vi "FPGAmain_5782_IQ_PID_2.vi"() -> ()   [LabVIEW 2018]
uses:
  FPGA/DataMode.ctl
  FPGA/Input_5782/5782_Fast_PID_states.ctl
  FPGA/Feed forward/FeedForwardState.ctl
  <vilib>/Platform/TimedLoop/XDataNode/timing_clust.ctl
  <vilib>/Platform/TimedLoop/XDataNode/nitl_modes.ctl
  <vilib>/Platform/TimedLoop/XDataNode/wakeup.ctl
  <vilib>/rvi/Emulation/niFpgaSctlEmulationGetInTimedLoop.vi
  <vilib>/rvi/Emulation/niFpgaEmulationReportErrorSimple.vi
  <vilib>/rvi/Emulation/niFpgaGetClockAttributes.vi
  <vilib>/rvi/Emulation/niFpgaCriticalErrorInLSC.vi
  <vilib>/rvi/Emulation/niFpgaProcessEmulError.vi
  <vilib>/rvi/Emulation/niFpgaEmulationIsFPGAContextNoSignature.vi
  <vilib>/rvi/errors/niFpgaSetErrorForExecOnDevCompSimple.vi
  <vilib>/rvi/eio/common/nirviEmuReportErrorAndStop.vi
  <vilib>/rvi/DataTransferAndStorage/Container/Common/niFpgaContainerGetUniqueNameForEmu.vi
  <vilib>/rvi/FIFO/Fifo_Resource/nirvififoEmulationSetSize.vi
  <vilib>/rvi/FIFO/Fifo_Resource/nirviFifoEmulationQueueMgr.vi
  <instcachedir>/0/nirviFifoEmulationQueueMgr_E5CAEC123FF24DC58D834DCA3CDAA9B5.lvgen/nirviFifoEmulationQueueMgr_E5CAEC123FF24DC58D834DCA3CDAA9B5_015.vi
  <vilib>/rvi/FIFO/Fifo_Resource/nirvififoEmulationDetermineInputValidOut.vi
  <vilib>/rvi/FIFO/Fifo_Resource/nirvififoEmulationCreateLock.vi
  <vilib>/rvi/FIFO/Fifo_Resource/nirvififoEmulationObtainLock.vi
  <vilib>/rvi/FIFO/Fifo_Resource/nirvififoEmulationReleaseLock.vi
  <vilib>/rvi/occurrence/nirviWaitOnOccurrenceBase.vi
  <vilib>/rvi/errors/nirviReportUnexpectedCaseInternalError.vi
  <vilib>/rvi/errors/nirviReportUnexpectedCaseInternalError (U32).vi
  <vilib>/rvi/Memory/Memory_Emulation/niFpgaMemoryEmulationCacheClearOnFirstRun.vi
  <vilib>/rvi/Memory/Memory_Emulation/nirvimemoryEmulationManagerCache_MakeExclusive.vi
  <vilib>/rvi/Memory/Memory_Emulation/niFpgaMemoryEmulationValidateCache.vi
  <vilib>/rvi/Memory/Memory_Emulation/nirvimemoryEmulationManagerCache_InsertValue.vi
  <vilib>/Utility/error.llb/Clear Errors.vi
  <vilib>/rvi/Memory/Memory_Emulation/nirvimemoryEmulationManagerCache_ReleaseExclusive.vi
  <vilib>/rvi/Memory/Memory_Emulation/nirvimemoryEmulationManagerCache_GetValue.vi
  <vilib>/rvi/Memory/Memory_Emulation/nirvimemoryEmulationManagerCache_SetValue.vi
  <vilib>/rvi/eio/common/nirviEmuTemplateMethod_errors.vi
  <instcachedir>/0/nirviFifoEmulationQueueMgr_E5CAEC123FF24DC58D834DCA3CDAA9B5.lvgen/nirviFifoEmulationQueueMgr_E5CAEC123FF24DC58D834DCA3CDAA9B5_018.vi
  <vilib>/rvi/interface/RandomDataEmulation/niFpgaRandomDataHandleErrors.vi
  <instcachedir>/0/nirviFifoEmulationQueueMgr_E5CAEC123FF24DC58D834DCA3CDAA9B5.lvgen/nirviFifoEmulationQueueMgr_E5CAEC123FF24DC58D834DCA3CDAA9B5_003.vi
  <instcachedir>/0/nirviFifoEmulationQueueMgr_E5CAEC123FF24DC58D834DCA3CDAA9B5.lvgen/nirviFifoEmulationQueueMgr_E5CAEC123FF24DC58D834DCA3CDAA9B5_017.vi
  <vilib>/rvi/interface/RandomDataEmulation/nirviRandomDataMultiElementFPGAFIFO.vi
  <instcachedir>/0/nirviRandomDataMultiElementFPGAFIFO_6740B454F3C245F78F76ED91F73FD8DB.lvgen/nirviRandomDataMultiElementFPGAFIFO_6740B454F3C245F78F76ED91F73FD8DB_000.vi
  <instrlib>/_niInstr/Basic Elements/v1/FPGA/Private/Count Down U8.vi
  <vilib>/rvi/Memory/Memory_Emulation/nirvimemoryFastEmulation.vi
  <vilib>/rvi/Memory/Memory_Emulation/nirvimemoryEmulation.vi
  <vilib>/Platform/TimedLoop/XDataNode/XDataNode.xnode
  <vilib>/rvi/FXPMathLib/FxpInterpret/XNode/nifxpmath_Interpret.xnode
  <vilib>/rvi/DataTransferAndStorage/Container/XNode/niFpgaContainer.xnode
  <vilib>/rvi/FIFO/Fifo_Resource/nirvififoEmulationWrite.vi
  <vilib>/rvi/DataTransferAndStorage/Register/Emulation/niFpgaRegisterEmulation.vi
  <vilib>/eio/EIONode/EIONode.xnode
  <vilib>/rvi/FIFO/Fifo_Resource/nirvififoEmulationRead.vi
  <vilib>/rvi/interface/RandomDataEmulation/nirviRandomDataFpgaReadWriteTemplate.vi
  <vilib>/rvi/interface/RandomDataEmulation/nirviRandomDataFpgaMultiElementTemplate.vi
  <vilib>/Platform/TimedLoop/XDataNode/XDNodeRunTimeDep.lvlib
  <instrlib>/_niInstr/Basic Elements/v1/FPGA/niInstr Basic Elements v1 FPGA.lvlib
panel:
  in  "Load FF":bool
  in  "Clear feedback buffers":bool
  in  "FF buffers manual":bool
  in  "Full speed transfer":bool
  in  "IO Module\\AO Data Sync":bool=TRUE
  in  "IO Module\\SPI Write Data":u16
  out "IO Module\\SPI Read Data":u8
  in  "IO Module\\SPI Read":bool
  in  "IO Module\\SPI Write":bool
  in  "IO Module\\SPI Address":u16
  in  "IO Module\\SPI Device":u8
  out "IO Module\\SPI Idle":bool
  in  "AM phase":fxp<+,64,64>
  in  "User Command Commit":bool
  in  "User Command":u8
  out "User Command Idle":bool
  out "User Command Status":u8
  in  "User Data 0":u8
  in  "User Data 1":u8
  out "PLL Locked":bool
  out "User Error":bool
  out "Configured?":bool
  in  "Continuous":bool
  in  "Record length":u16=4000 caption="Samples Per Trigger" min=1 step=1
  in  "Trigger Acquisition":bool
  out "IO Module\\Trigger Input":bool
  in  "Acquisition running":bool
  in  "Phase output":fxp<+,64,64>[](array[numeric])=[0.0, 0.0, 0.0, 0.0]
  in  "Simulated phase":fxp<+,64,64>[](array[numeric])=[0.0, 0.0]
  in  "Mode":T1
  in  "Phase input":fxp<+,64,64>[](array[numeric])=[0.0, 0.0, 0.0, 0.0, 0.0, 0.0, 0.0, 0.0, 0.0, 0.0, 0.0, 0.0, 0.0, 0.0, 0.0, 0.0]
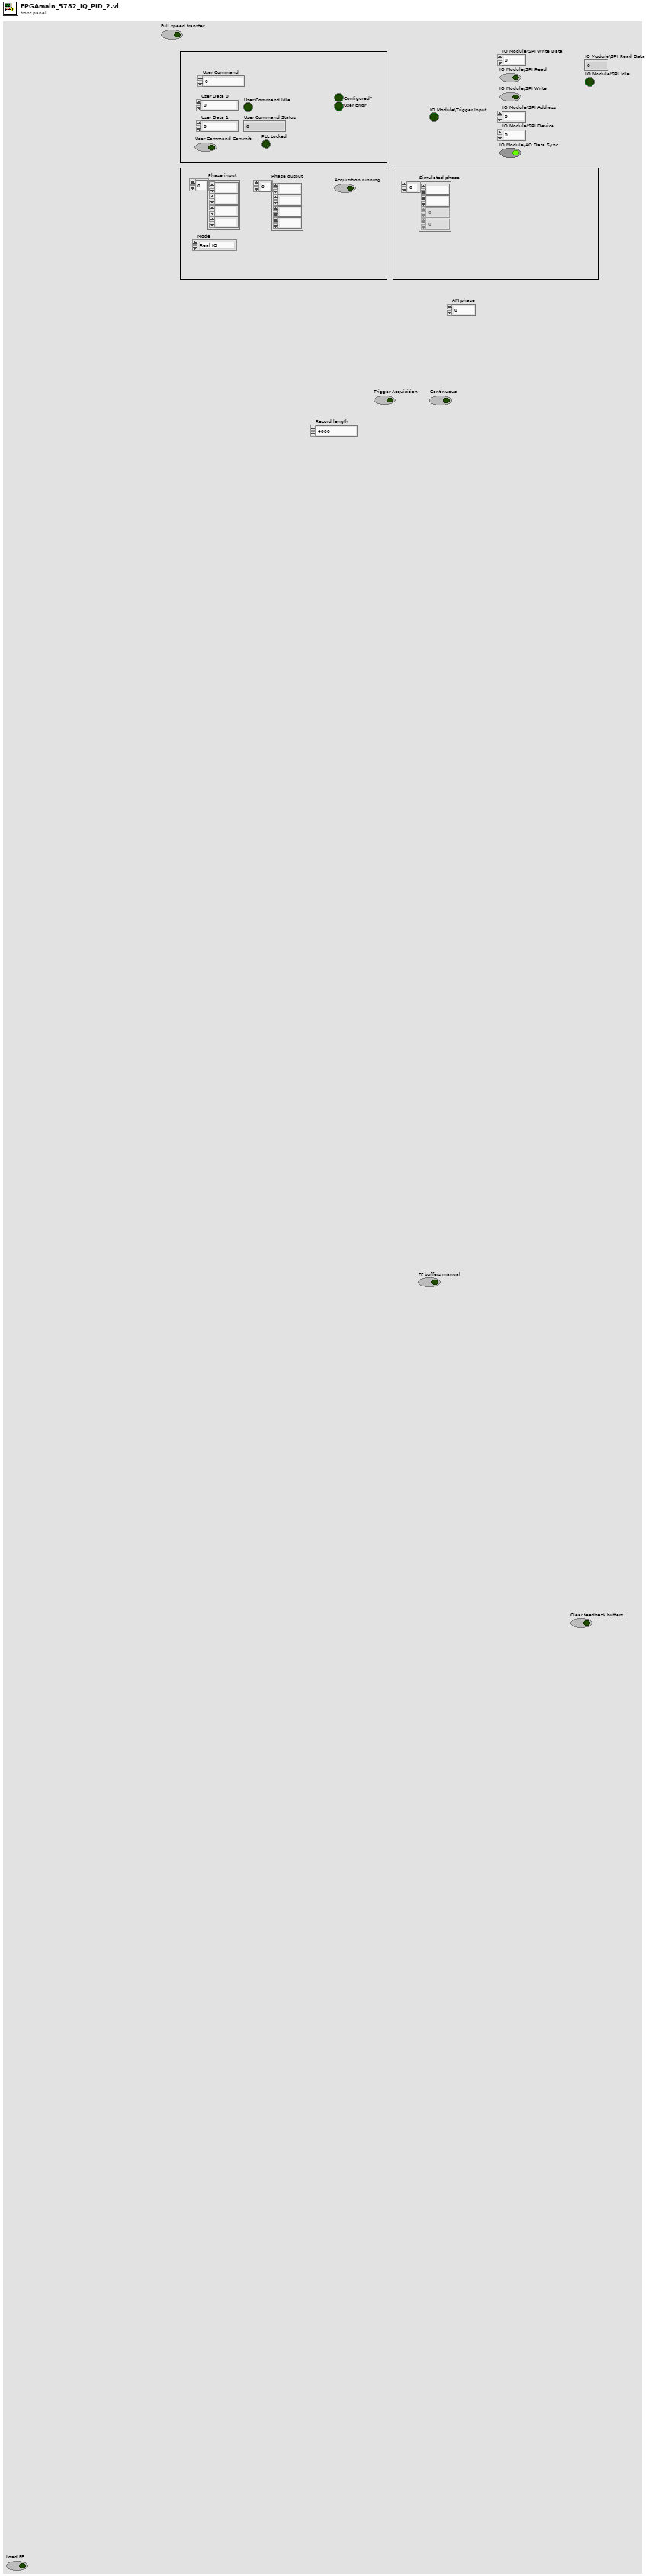
[diagram p1: front panel]
types:
  T1 = typedef "DataMode.ctl" = enum16{"Real IO", "Simulated"}
  T2 = typedef "FeedForwardState.ctl" = enum16{"Idle", "Wait for trigger", "Read FF", "Clear FF", "Wait for reset"}
  T3 = typedef "5782_Fast_PID_states.ctl" = enum8{"Wait for trigger", "Acquisition", "Send record length", "Wait for output", "Quiet period"}
  T4 = typedef "XDNodeRunTimeDep.lvlib/timing_clust.ctl" = cluster{"Expected End [f-1]":u64, "Actual End [f-1]":u64, "Finished Late? [f-1]":bool, "Expected End [i-1]":u64, "Actual End [i-1]":u64, "Finished Late? [i-1]":bool, "Expected Start [i]":u64, "Actual Start [i]":u64, "Expected Start [f]":u64, "Actual Start [f]":u64, "Source Name":string, "Structure Name":string, "Period":i64, "Deadline":i64, "Offset":i64, "Start":i64, "Priority":i32, "Timeout":i32, "Mode":T5, "Wakeup Reason":T6, "Error":errorcluster, "Source Type":string, "Secondary Source Type":string, "Global End Time":u64, "Global Start Time":u64, "Frame Duration":u64, "Iteration Duration":u64, "Assigned CPU":i32, "I/O Scan Engine Mode":u32}
  T5 = typedef "XDNodeRunTimeDep.lvlib/nitl_modes.ctl" = enum32{"No Change", "Process missed periods, maintain original phase", "Discard missed periods, maintain original phase", "Process missed periods, ignore original phase", "Discard missed periods, ignore original phase"}
  T6 = typedef "XDNodeRunTimeDep.lvlib/wakeup.ctl" = enum32{"Normal", "Aborted", "Asynchronous wakeup", "Timing source error", "Timed loop error", "Timeout"}
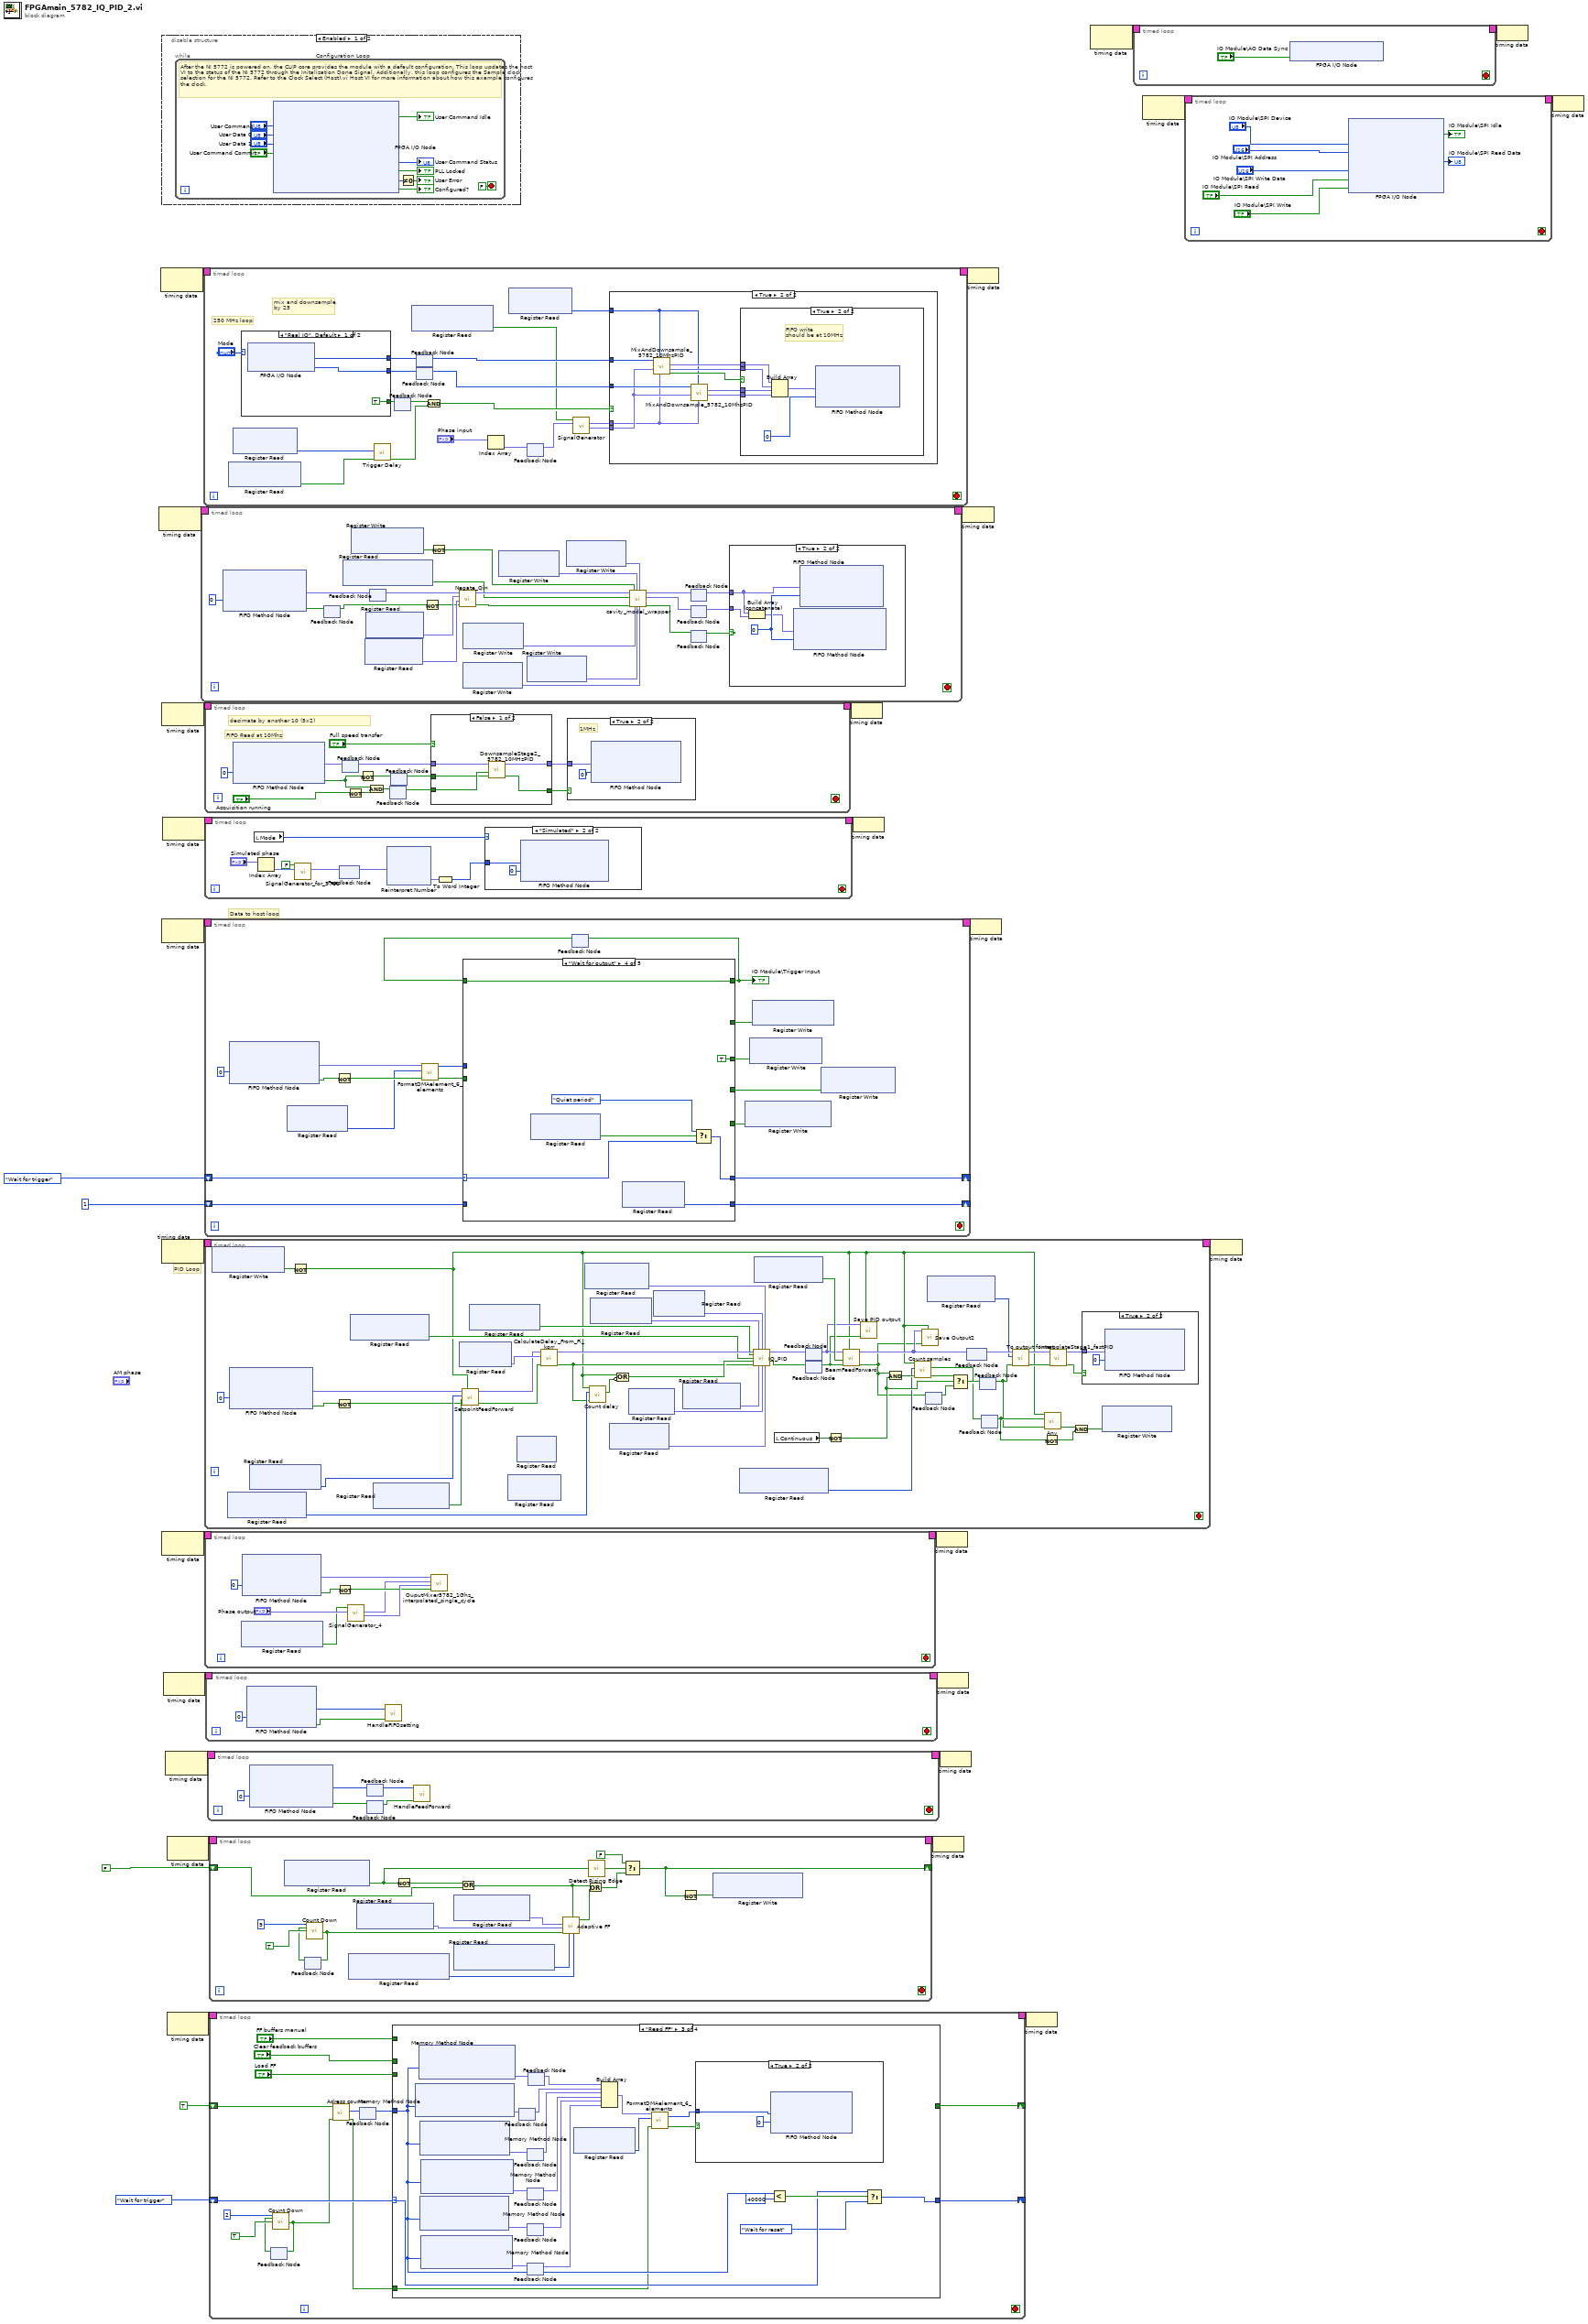
[diagram p0: block diagram]
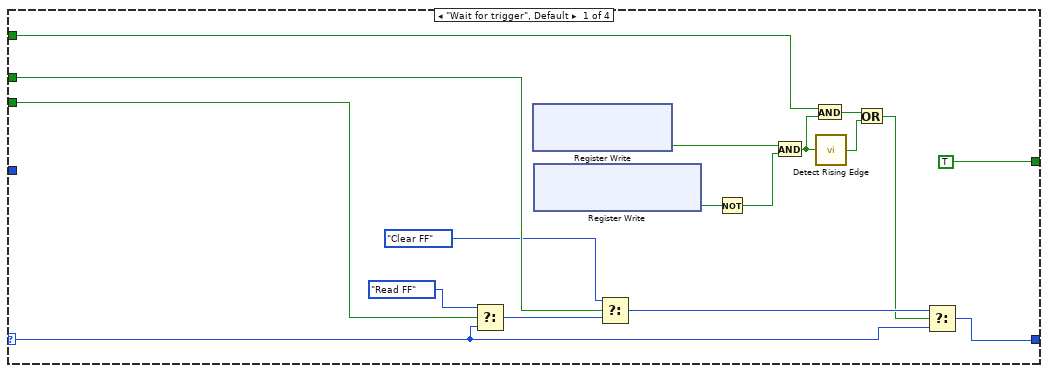
[diagram p2: hidden frame]
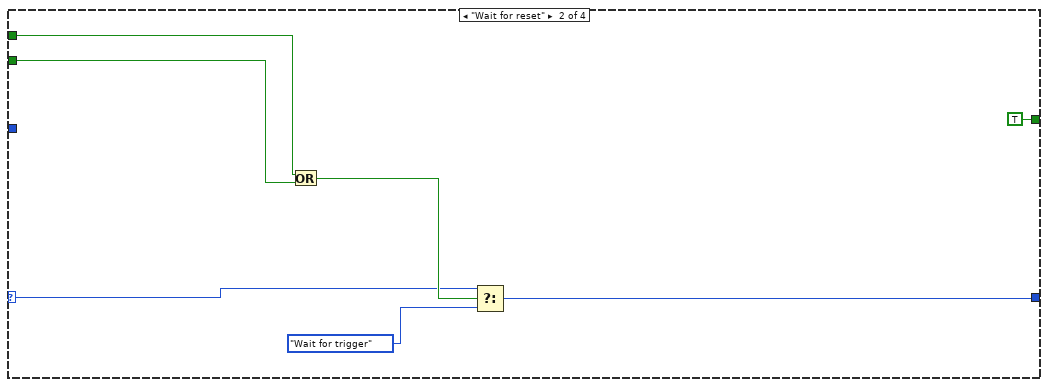
[diagram p3: hidden frame]
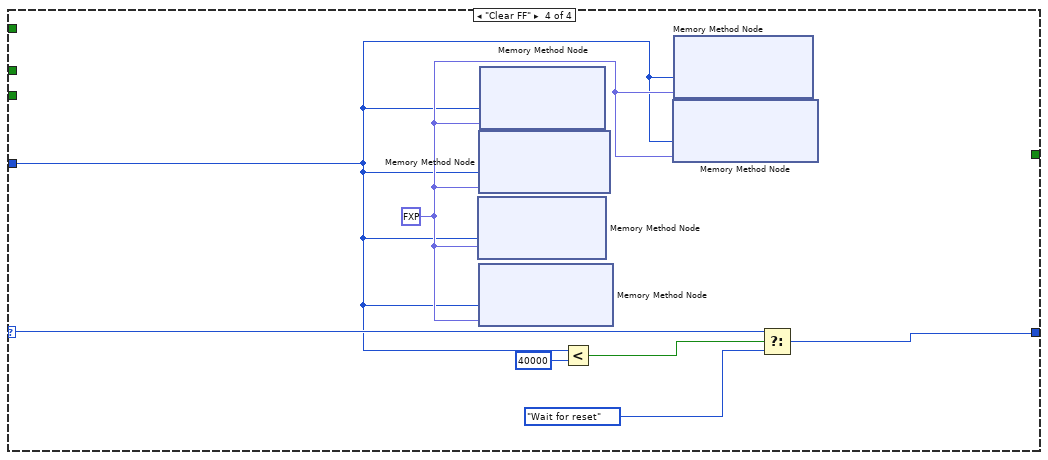
[diagram p5: hidden frame]
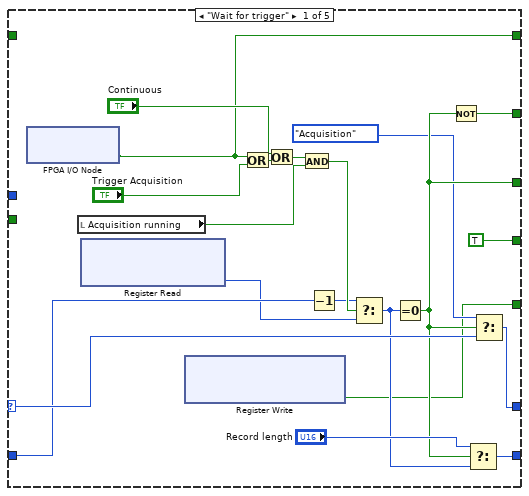
[diagram p7: hidden frame]
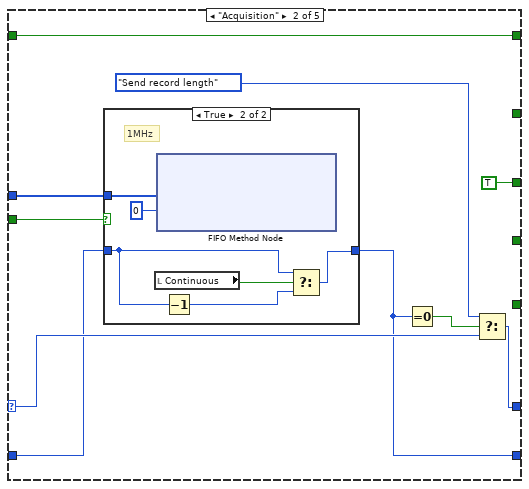
[diagram p8: hidden frame]
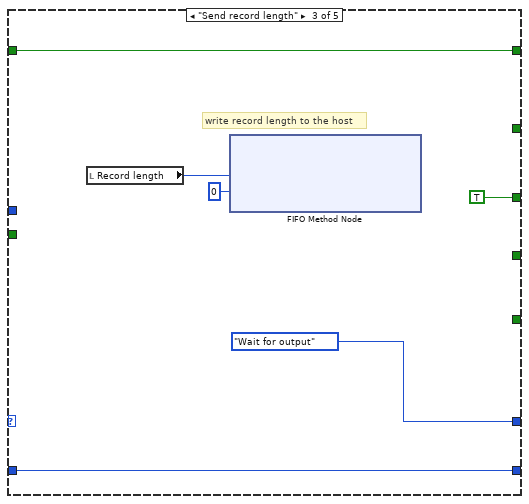
[diagram p10: hidden frame]
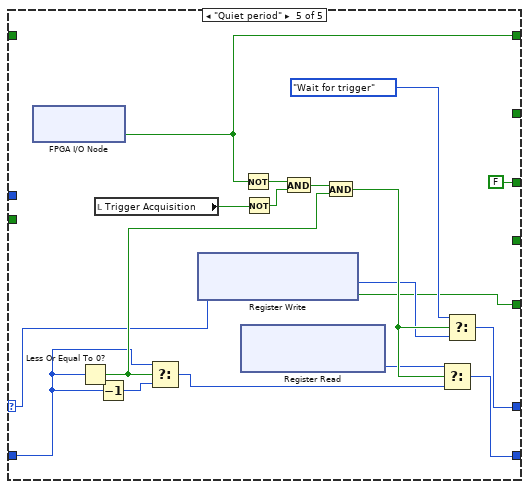
[diagram p11: hidden frame]
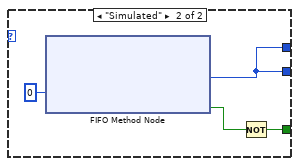
[diagram p18: hidden frame]
diagram:
  # "PID Loop"
  # "Data to host loop"
  n1 = node-c288() -> (w9:T4)  [unwired: 1 in]
  n2 = node-c288() -> (w29:T4)  [unwired: 1 in]
  n3 = disable-structure shown="Enabled" {
    frame Enabled {
      n4 = while "Configuration Loop" {
        stop <- FALSE stop-if-true
        # "After the NI 5772 is powered on, the CLIP core provides the module with a default configuration. This loop updates the host VI to the status of the NI 5772 through the Initalization Done Signal. Additionally, this loop configures the Sample clock selection for the NI 5772. Refer to the Clock Select (Host).vi Host VI for more information about how this example configures the clock."
        n5 = xnode "FPGA I/O Node"("IO Module\\User Command"="User Command", "IO Module\\User Data 0"="User Data 0", "IO Module\\User Data 1"="User Data 1", "IO Module\\User Command Commit"="User Command Commit") -> ("IO Module\\User Command Idle"=→"User Command Idle":bool, "IO Module\\User Command Status"=→"User Command Status":u8, "IO Module\\PLL Locked"=→"PLL Locked":bool, "IO Module\\User Error"=w37:u8, "IO Module\\Initialization Done"=→"Configured?":bool)  [unwired: 9 in, 9 out]
        n6 = Not Equal To 0?(x=w37) -> (x != 0?=→"User Error":bool)
      }
    }
    frame Disabled {
    }
  }
  n7 = node-c288() -> (w16:T4)  [unwired: 1 in]
  n8 = node-c288() -> (w14:T4)  [unwired: 1 in]
  n9 = node-c288() -> (w18:T4)  [unwired: 1 in]
  n10 = node-c288() -> (w24:T4)  [unwired: 1 in]
  n11 = node-c288() -> (w31:T4)  [unwired: 1 in]
  n12 = node-c288() -> (w26:T4)  [unwired: 1 in]
  n13 = node-c288() -> (w11:T4)  [unwired: 1 in]
  n14 = node-c288() -> (w7:T4)  [unwired: 1 in]
  n15 = node-c288() -> (w5:T4)  [unwired: 1 in]
  n16 = timed-loop {
    timing: w9 -> [_]
    timing-out: [_] -> w8
    stop <- _ stop-if-true
    n17 = xnode ("FIFO Method Node")("Timeout"=0) -> ("Element"=w52:fxp<+/-,32,14>[], "Timed Out?"=w51:bool)  [unwired: 1 in, 1 out]
    n18 = feedback #1() -> (w49:bool)  [unwired: 1 in]
    n19 = feedback-in #1(w51) -> ()
    n20 = xnode ("Register Read")() -> ("Data"=w60:bool)  [unwired: 1 in, 1 out]
    n21 = xnode ("Register Write")() -> ("Data"=w59:bool)  [unwired: 1 in, 1 out]
    n22 = xnode ("Register Read")() -> ("Data"=w65:fxp<+/-,32,14>)  [unwired: 1 in, 1 out]
    n23 = xnode ("Register Read")() -> ("Data"=w66:fxp<+/-,32,14>)  [unwired: 1 in, 1 out]
    n24 = feedback #2() -> (w50:fxp<+/-,32,14>[])  [unwired: 1 in]
    n25 = feedback-in #2(w52) -> ()
    n26 = Not(x=w49) -> (.not. x?=w64:bool)
    n27 = Not(x=w59) -> (.not. x?=w61:bool)
    n28 = call "Negate_Qin.vi"("valid in"=w64, "DC offset chan 1"=w65, "DC offset chan 0"=w66, "Data in"=w50) -> ("valid out"=w62:bool, "Data out"=w63:fxp<+/-,32,14>[])  [unwired: 6 in]
    n29 = xnode ("Register Write")() -> ("Data"=w45:fxp<+/-,32,-32>)  [unwired: 1 in, 1 out]
    n30 = xnode ("Register Write")() -> ("Data"=w43:fxp<+/-,32,3>)  [unwired: 1 in, 1 out]
    n31 = xnode ("Register Write")() -> ("Data"=w46:fxp<+/-,32,1>)  [unwired: 1 in, 1 out]
    n32 = xnode ("Register Write")() -> ("Data"=w44:fxp<+/-,32,1>)  [unwired: 1 in, 1 out]
    n33 = xnode ("Register Write")() -> ("Data"=w47:fxp<+/-,32,3>)  [unwired: 1 in, 1 out]
    n34 = call "cavity_model_wrapper.vi"("Data in"=w63, "enabled"=w60, "input valid"=w62, "reset"=w61, "C3"=w43, "C1"=w46, "C4"=w44, "C2"=w47, "C5"=w45) -> ("Data out"=w58:fxp<+/-,32,14>[], "Ai1 out"=w54:fxp<+/-,32,14>[], "output valid"=w56:bool)  [unwired: 8 in]
    n35 = feedback #3() -> (w57:fxp<+/-,32,14>[])  [unwired: 1 in]
    n36 = feedback-in #3(w58) -> ()
    n37 = feedback #4() -> (w53:fxp<+/-,32,14>[])  [unwired: 1 in]
    n38 = feedback-in #4(w54) -> ()
    n39 = feedback #5() -> (w55:bool)  [unwired: 1 in]
    n40 = feedback-in #5(w56) -> ()
    n41 = case shown="True" w55 {
      tunnel: w57 -> [_ w69]
      tunnel: w53 -> [_ w68]
      frame False {
      }
      frame True {
        w70 = 0 ("Timeout")
        n42 = Build Array (concatenate)(w69, w68) -> (w67:fxp<+/-,32,14>[])
        n43 = xnode ("FIFO Method Node")("Element"=w67, "Timeout"=w70) -> ()  [unwired: 1 in, 2 out]
        n44 = xnode ("FIFO Method Node")("Element"=w69, "Timeout"=w70) -> ()  [unwired: 1 in, 2 out]
      }
    }
  }
  n45 = timed-loop {
    timing: w29 -> [_]
    timing-out: [_] -> w28
    stop <- _ stop-if-true
    # "mix and downsample\nby 25"
    # "250 MHz loop"
    n46 = xnode ("Register Read")() -> ("Data"=w76:bool)  [unwired: 1 in, 1 out]
    n47 = xnode ("Register Read")() -> ("Data"=w74:u32)  [unwired: 1 in, 1 out]
    n48 = case shown="\"Real IO\", Default" "Mode" {
      tunnel: [w109 w110] -> w89
      tunnel: [w108 w110] -> w87
      tunnel: [TRUE w111] -> w85
      frame "Real IO", Default {
        n49 = xnode "FPGA I/O Node"() -> ("IO Module\\AI 0"=w109:i16, "IO Module\\AI 1"=w108:i16)  [unwired: 2 in, 2 out]
      }
      frame "Simulated" {
        n50 = xnode ("FIFO Method Node")("Timeout"=0) -> ("Element"=w110:i16, "Timed Out?"=w112:bool)  [unwired: 1 in, 1 out]
        n51 = Not(x=w112) -> (.not. x?=w111:bool)
      }
    }
    n52 = call "Trigger Delay.vi"("input valid"=w76, "Count to skip"=w74) -> ("output valid"=w75:bool)  [unwired: 9 in]
    n53 = feedback #6() -> (w84:bool)  [unwired: 1 in]
    n54 = feedback-in #6(w85) -> ()
    n55 = xnode ("Register Read")() -> ("Data"=w80:bool)  [unwired: 1 in, 1 out]
    n56 = feedback #7() -> (w88:i16)  [unwired: 1 in]
    n57 = feedback-in #7(w89) -> ()
    n58 = feedback #8() -> (w86:i16)  [unwired: 1 in]
    n59 = feedback-in #8(w87) -> ()
    n60 = And(x=w84, y=w75) -> (x .and. y?=w81:bool)
    n61 = Index Array(array="Phase input") -> (element=w78:fxp<+,64,64>)  [unwired: 1 in]
    n62 = xnode ("Register Read")() -> ("Data"=w73:u16)  [unwired: 1 in, 1 out]
    n63 = feedback #9() -> (w77:fxp<+,64,64>)  [unwired: 1 in]
    n64 = feedback-in #9(w78) -> ()
    n65 = call "SignalGenerator.vi"("phase"=w77, "Reset"=w80) -> ("Cos"=w83:fxp<+/-,16,0>, "Sin"=w82:fxp<+/-,16,0>)  [unwired: 7 in, 1 out]
    n66 = case shown="True" w81 {
      tunnel: w88 -> [_ w100]
      tunnel: w86 -> [_ w99]
      tunnel: w83 -> [_ w93]
      tunnel: w82 -> [_ w92]
      tunnel: w73 -> [_ w91]
      frame False {
      }
      frame True {
        n67 = call "MixAndDownsample_5782_10MhzPID.vi"("sin0"=w92, "factor"=w91, "cos0"=w93, "signal 0"=w100) -> ("data valid"=w96:bool, "Q out"=w97:fxp<+/-,32,14>, "I out"=w98:fxp<+/-,32,14>)  [unwired: 5 in]
        n68 = call "MixAndDownsample_5782_10MhzPID.vi"("sin0"=w92, "factor"=w91, "cos0"=w93, "signal 0"=w99) -> ("Q out"=w94:fxp<+/-,32,14>, "I out"=w95:fxp<+/-,32,14>)  [unwired: 5 in, 1 out]
        n69 = case shown="True" w96 {
          tunnel: w97 -> [_ w106]
          tunnel: w98 -> [_ w105]
          tunnel: w95 -> [_ w104]
          tunnel: w94 -> [_ w103]
          frame False {
          }
          frame True {
            # "FIFO write\nshould be at 10MHz"
            n70 = Build Array(w105, w106, w104, w103) -> (w102:fxp<+/-,32,14>[])
            n71 = xnode ("FIFO Method Node")("Element"=w102, "Timeout"=0) -> ()  [unwired: 1 in, 2 out]
          }
        }
      }
    }
  }
  n72 = timed-loop {
    timing: w16 -> [_]
    timing-out: [_] -> w15
    stop <- _ stop-if-true
    # "FIFO Read at 10Mhz"
    # "decimate by another 10 (5x2)"
    n73 = xnode ("FIFO Method Node")("Timeout"=0) -> ("Element"=w124:fxp<+/-,32,14>[], "Timed Out?"=w125:bool)  [unwired: 1 in, 1 out]
    n74 = feedback #10() -> (w123:fxp<+/-,32,14>[])  [unwired: 1 in]
    n75 = feedback-in #10(w124) -> ()
    n76 = Not(x="Acquisition running") -> (.not. x?=w117:bool)
    n77 = Not(x=w125) -> (.not. x?=w119:bool)
    n78 = And(x=w125, y=w117) -> (x .and. y?=w121:bool)
    n79 = feedback #11() -> (w120:bool)  [unwired: 1 in]
    n80 = feedback-in #11(w121) -> ()
    n81 = feedback #12() -> (w118:bool)  [unwired: 1 in]
    n82 = feedback-in #12(w119) -> ()
    n83 = case shown="False" "Full speed transfer" {
      tunnel: [w133 w135] -> w127
      tunnel: [w132 w134] -> w126
      tunnel: w123 -> [w131 w135]
      tunnel: w120 -> [w130 _]
      tunnel: w118 -> [w129 w134]
      frame False {
        n84 = call "DownsampleStage2_5782_10MHzPID.vi"("valid in"=w129, "reset"=w130, "Data in"=w131) -> ("valid out"=w132:bool, "data out"=w133:fxp<+/-,32,14>[])  [unwired: 7 in]
      }
      frame True {
      }
    }
    n85 = case shown="True" w126 {
      tunnel: w127 -> [_ w136]
      frame False {
      }
      frame True {
        # "1MHz"
        n86 = xnode ("FIFO Method Node")("Element"=w136, "Timeout"=0) -> ()  [unwired: 1 in, 2 out]
      }
    }
  }
  n87 = timed-loop {
    timing: w14 -> [_]
    timing-out: [_] -> w13
    shift-right: [w154] -> _
    shift-left: 5782_Fast_PID_states."Wait for trigger" ("5782 states") -> [w156]
    shift-right: [w153] -> _
    shift-left: u16 1 ("trigger samples") -> [w155]
    stop <- _ stop-if-true
    n88 = xnode ("FIFO Method Node")("Timeout"=0) -> ("Element"=w144:fxp<+/-,32,14>[], "Timed Out?"=w151:bool)  [unwired: 1 in, 1 out]
    n89 = xnode ("Register Read")() -> ("Data"=w142:u16)  [unwired: 1 in, 1 out]
    n90 = Not(x=w151) -> (.not. x?=w143:bool)
    n91 = call "FormatDMAelement_6_elements.vi"("valid in"=w143, "factor"=w142, "Data in"=w144) -> ("valid out"=w147:bool, "Values"=w146:u64[])  [unwired: 7 in]
    n92 = feedback #13() -> (w149:bool)  [unwired: 1 in]
    n93 = case shown="\"Wait for output\"" w156 {
      selector: w156 -> [w176 w186 _ w204 w210]
      tunnel: w155 -> [w167 w183 w194 _ w211]
      tunnel: [w175 w185 5782_Fast_PID_states."Wait for output" ("5782 states") w206 w222] -> w154
      tunnel: [w174 w180 w194 w202 w223] -> w153
      tunnel: w146 -> [_ w181 _ _ _]
      tunnel: w147 -> [_ w182 _ _ _]
      tunnel: [w162 TRUE TRUE ("5782 triggered") TRUE ("5782 triggered") FALSE ("5782 triggered")] -> w150
      tunnel: [w159 w179 w196 w200 w208] -> w148
      tunnel: w149 -> [_ w179 w196 w200 _]
      tunnel: [w161 _ _ _ _] -> w145
      tunnel: [TRUE _ _ _ _] -> w141
      tunnel: [w158 _ _ _ w207] -> w140
      frame "Wait for trigger" {
        n94 = xnode "FPGA I/O Node"() -> ("PXI_Trig0"=w159:bool)  [unwired: 1 in, 1 out]
        n95 = local read "Acquisition running"() -> (w170:bool)
        n96 = xnode ("Register Read")() -> ("Data"=w163:u16)  [unwired: 1 in, 1 out]
        n97 = xnode ("Register Write")() -> ("Data"=w158:bool)  [unwired: 1 in, 1 out]
        n98 = Or(x=w159, y="Trigger Acquisition") -> (x .or. y?=w166:bool)
        n99 = Or(x="Continuous", y=w166) -> (x .or. y?=w164:bool)
        n100 = And(x=w164, y=w170) -> (x .and. y?=w171:bool)
        n101 = Decrement(x=w167) -> (x-1=w168:u16)
        n102 = Select(t=w168, s=w171, f=w163) -> (s? t:f=w169:u16)
        n103 = Equal To 0?(x=w169) -> (x = 0?=w162:bool)
        n104 = Not(x=w162) -> (.not. x?=w161:bool)
        n105 = Select(t="Record length", s=w162, f=w169) -> (s? t:f=w174:u16)
        n106 = Select(t=5782_Fast_PID_states."Acquisition" ("5782 states"), s=w162, f=w176) -> (s? t:f=w175:T3)
      }
      frame "Acquisition" {
        n107 = case shown="True" w182 {
          tunnel: w181 -> [_ w193]
          tunnel: [w187 w190] -> w180
          tunnel: w183 -> [w187 w188]
          frame False {
          }
          frame True {
            # "1MHz"
            n108 = local read "Continuous"() -> (w191:bool)
            n109 = xnode ("FIFO Method Node")("Element"=w193, "Timeout"=0) -> ()  [unwired: 1 in, 2 out]
            n110 = Decrement(x=w188) -> (x-1=w189:u16)
            n111 = Select(t=w188, s=w191, f=w189) -> (s? t:f=w190:u16)
          }
        }
        n112 = Equal To 0?(x=w180) -> (x = 0?=w184:bool)
        n113 = Select(t=5782_Fast_PID_states."Send record length" ("5782 states"), s=w184, f=w186) -> (s? t:f=w185:T3)
      }
      frame "Send record length" {
        # "write record length to the host"
        n114 = local read "Record length"() -> (w198:u16)
        n115 = xnode ("FIFO Method Node")("Element"=w198, "Timeout"=0) -> ()  [unwired: 1 in, 2 out]
      }
      frame "Wait for output" {
        n116 = xnode ("Register Read")() -> ("Data"=w201:bool)  [unwired: 1 in, 1 out]
        n117 = xnode ("Register Read")() -> ("Data"=w202:u16)  [unwired: 1 in, 1 out]
        n118 = Select(t=5782_Fast_PID_states."Quiet period" ("5782 states"), s=w201, f=w204) -> (s? t:f=w206:T3)
      }
      frame "Quiet period" {
        n119 = xnode "FPGA I/O Node"() -> ("PXI_Trig0"=w208:bool)  [unwired: 1 in, 1 out]
        n120 = Less Or Equal To 0?(x=w211) -> (x <= 0?=w214:bool)
        n121 = local read "Trigger Acquisition"() -> (w220:bool)
        n122 = Decrement(x=w211) -> (x-1=w215:u16)
        n123 = Select(t=w211, s=w214, f=w215) -> (s? t:f=w213:u16)
        n124 = xnode ("Register Write")() -> ("Data"=w207:bool)  [unwired: 1 in, 1 out]
        n125 = xnode ("Register Read")() -> ("Data"=w212:u16)  [unwired: 1 in, 1 out]
        n126 = Not(x=w208) -> (.not. x?=w219:bool)
        n127 = Not(x=w220) -> (.not. x?=w218:bool)
        n128 = And(x=w219, y=w218) -> (x .and. y?=w217:bool)
        n129 = And(x=w217, y=w214) -> (x .and. y?=w221:bool)
        n130 = Select(t=w212, s=w221, f=w213) -> (s? t:f=w223:u16)
        n131 = Select(t=5782_Fast_PID_states."Wait for trigger" ("5782 states"), s=w221, f=w210) -> (s? t:f=w222:T3)
      }
    }
    "IO Module\\Trigger Input" <- w148
    n132 = feedback-in #13(w148) -> ()
    n133 = xnode ("Register Write")("Data"=w140) -> ()  [unwired: 1 in, 1 out]
    n134 = xnode ("Register Write")("Data"=w150) -> ()  [unwired: 1 in, 1 out]
    n135 = xnode ("Register Write")("Data"=w145) -> ()  [unwired: 1 in, 1 out]
    n136 = xnode ("Register Write")("Data"=w141) -> ()  [unwired: 1 in, 1 out]
  }
  n137 = timed-loop {
    timing: w18 -> [_]
    timing-out: [_] -> w17
    stop <- _ stop-if-true
    n138 = xnode ("Register Write")() -> ("Data"=w273:bool)  [unwired: 1 in, 1 out]
    n139 = xnode ("Register Read")() -> ("Data"=w268:u32)  [unwired: 1 in, 1 out]
    n140 = xnode ("FIFO Method Node")("Timeout"=0) -> ("Element"=w266:fxp<+/-,32,14>[], "Timed Out?"=w274:bool)  [unwired: 1 in, 1 out]
    n141 = xnode ("Register Read")() -> ("Data"=w267:u32)  [unwired: 1 in, 1 out]
    n142 = Not(x=w273) -> (.not. x?=w227:bool)
    n143 = Not(x=w274) -> (.not. x?=w265:bool)
    n144 = xnode ("Register Read")() -> ("Data"=w252:bool)  [unwired: 1 in, 1 out]
    n145 = xnode ("Register Read")() -> ("Data"=w272:bool)  [unwired: 1 in, 1 out]
    n146 = xnode ("Register Read")() -> ("Data"=w264:fxp<+/-,32,4>)  [unwired: 1 in, 1 out]
    n147 = call "SetpointFeedForward.vi"("Reset"=w227, "input valid"=w265, "setpoint enabled"=w272, "Samples to skip"=w267, "Data in"=w266) -> ("output valid"=w263:bool, "Data out"=w262:fxp<+/-,32,14>[])  [unwired: 5 in]
    n148 = xnode ("Register Read")() -> ("Data"=w260:bool)  [unwired: 1 in, 1 out]
    n149 = xnode ("Register Read")() -> ()  [unwired: 1 in, 2 out]
    n150 = xnode ("Register Read")() -> ()  [unwired: 1 in, 2 out]
    n151 = call "CalculateDelay_From_Fi_korr.vi"("input valid"=w263, "fi_korr"=w264, "Data in"=w262) -> ("output valid"=w253:bool, "Data out"=w261:fxp<+/-,32,14>[])  [unwired: 7 in]
    n152 = xnode ("Register Read")() -> ("Data"=w255:fxp<+/-,32,6>)  [unwired: 1 in, 1 out]
    n153 = call "Count delay.vi"("input valid"=w253, "Count to skip"=w268, "Reset"=w227) -> ("count done?"=w269:bool)  [unwired: 7 in, 1 out]
    n154 = xnode ("Register Read")() -> ("Data"=w259:fxp<+/-,32,6>)  [unwired: 1 in, 1 out]
    n155 = xnode ("Register Read")() -> ("Data"=w249:fxp<+/-,32,6>)  [unwired: 1 in, 1 out]
    n156 = Compound Arithmetic op=OR(w227, invert w269) -> (w254:bool)
    n157 = xnode ("Register Read")() -> ("Data"=w250:fxp<+/-,32,6>)  [unwired: 1 in, 1 out]
    n158 = xnode ("Register Read")() -> ("Data"=w258:fxp<+/-,32,6>)  [unwired: 1 in, 1 out]
    n159 = xnode ("Register Read")() -> ("Data"=w251:fxp<+/-,32,6>)  [unwired: 1 in, 1 out]
    n160 = xnode ("Register Read")() -> ("Data"=w238:u32)  [unwired: 1 in, 1 out]
    n161 = call "IQ_PID.vi"("Data in"=w261, "Ki*Tau I"=w259, "Kp I"=w258, "Kd/Tau I"=w255, "Enable I"=w260, "Enable Q"=w252, "Reset"=w254, "input valid"=w253, "Ki*Tau Q"=w251, "Kp Q"=w250, "Kd/Tau Q"=w249) -> ("data out"=w257:fxp<+/-,32,14>[], "output valid"=w256:bool)  [unwired: 3 in]
    n162 = xnode ("Register Read")() -> ("Data"=w271:bool)  [unwired: 1 in, 1 out]
    n163 = local read "Continuous"() -> (w248:bool)
    n164 = feedback #14() -> (w230:fxp<+/-,32,14>[])  [unwired: 1 in]
    n165 = feedback-in #14(w257) -> ()
    n166 = feedback #15() -> (w229:bool)  [unwired: 1 in]
    n167 = feedback-in #15(w256) -> ()
    n168 = Not(x=w248) -> (.not. x?=w240:bool)
    n169 = call "BeamFeedForward.vi"("Reset"=w227, "input valid"=w229, "beam enabled"=w271, "Data in"=w230) -> ("output valid"=w226:bool, "Data out"=w228:fxp<+/-,32,14>[])  [unwired: 6 in]
    n170 = call "Save PID output.vi"("Reset"=w227, "input valid"=w229, "Data in"=w230) -> ()  [unwired: 9 in]
    n171 = And(x=w226, y=w240) -> (x .and. y?=w242:bool)
    n172 = call "Count samples.vi"("input valid"=w242, "number to count"=w238, "Reset"=w227) -> ("output valid"=w243:bool, "counting"=w239:bool)  [unwired: 7 in]
    n173 = call "Save Output2.vi"("Reset"=w227, "input valid"=w226, "Data in"=w228) -> ()  [unwired: 9 in]
    n174 = feedback #16() -> (w241:bool)  [unwired: 1 in]
    n175 = feedback-in #16(w226) -> ()
    n176 = xnode ("Register Read")() -> ("Data"=w231:u16)  [unwired: 1 in, 1 out]
    n177 = Select(t=w243, s=w240, f=w241) -> (s? t:f=w244:bool)
    n178 = feedback #17() -> (w235:fxp<+/-,32,14>[])  [unwired: 1 in]
    n179 = feedback-in #17(w228) -> ()
    n180 = feedback-in #18(w244) -> ()
    n181 = feedback #18() -> (w233:bool)  [unwired: 1 in]
    n182 = feedback #19() -> (w246:bool)  [unwired: 1 in]
    n183 = feedback-in #19(w239) -> ()
    n184 = call "To output format.vi"("input valid"=w233, "factor"=w231, "Data in"=w235) -> ("output valid"=w232:bool, "Data out"=w234:fxp<+/-,16,14>[])  [unwired: 7 in]
    n185 = Not(x=w246) -> (.not. x?=w245:bool)
    n186 = call "Any.vi"("input valid"=w233, "Value"=w246, "Reset"=w227) -> ("output valid"=w247:bool)  [unwired: 7 in, 1 out]
    n187 = call "InterpolateStage1_fastPID.vi"("valid in"=w232, "Data in"=w234) -> ("valid out"=w236:bool, "Data out"=w237:fxp<+/-,16,14>[])  [unwired: 8 in]
    n188 = And(x=w247, y=w245) -> (x .and. y?=w270:bool)
    n189 = case shown="True" w236 {
      tunnel: w237 -> [_ w277]
      frame False {
      }
      frame True {
        n190 = xnode ("FIFO Method Node")("Element"=w277, "Timeout"=0) -> ()  [unwired: 1 in, 2 out]
      }
    }
    n191 = xnode ("Register Write")("Data"=w270) -> ()  [unwired: 1 in, 1 out]
  }
  n192 = timed-loop {
    timing: w24 -> [_]
    timing-out: [_] -> w23
    stop <- _ stop-if-true
    n193 = xnode ("Register Read")() -> ("Data"=w280:bool)  [unwired: 1 in, 1 out]
    n194 = xnode ("FIFO Method Node")("Timeout"=0) -> ("Element"=w283:fxp<+/-,16,14>[], "Timed Out?"=w286:bool)  [unwired: 1 in, 1 out]
    n195 = Not(x=w286) -> (.not. x?=w282:bool)
    n196 = call "SignalGenerator_4.vi"("Phase"="Phase output", "reset"=w280) -> ("Sine out"=w284:fxp<+/-,16,0>[], "Cosine out"=w281:fxp<+/-,16,0>[])  [unwired: 8 in]
    n197 = call "OuputMixer5782_1Ghz_interpolated_single_cycle.vi"("input valid"=w282, "Sine in"=w284, "Cosine in"=w281, "Data"=w283) -> ()  [unwired: 7 in, 1 out]
  }
  n198 = timed-loop {
    timing: w31 -> [_]
    timing-out: [_] -> w30
    stop <- _ stop-if-true
    n199 = local read "Mode"() -> (w297:T1)
    n200 = Index Array(array="Simulated phase") -> (element=w296:fxp<+,64,64>)  [unwired: 1 in]
    n201 = call "SignalGenerator_for_5761.vi"("phase"=w296, "Reset"=FALSE) -> ("Sin"=w292:fxp<+/-,16,0>)  [unwired: 7 in, 2 out]
    n202 = feedback #20() -> (w293:fxp<+/-,16,0>)  [unwired: 1 in]
    n203 = feedback-in #20(w292) -> ()
    n204 = xnode "Reinterpret Number"("x"=w293) -> ("y"=w294:fxp<+/-,16,13>)
    n205 = To Word Integer(number=w294) -> (16bit integer=w290:i16)
    n206 = case shown="\"Simulated\"" w297 {
      tunnel: w290 -> [_ w298]
      frame "Real IO", Default {
      }
      frame "Simulated" {
        n207 = xnode ("FIFO Method Node")("Element"=w298, "Timeout"=0) -> ()  [unwired: 1 in, 2 out]
      }
    }
  }
  n208 = timed-loop {
    timing: w26 -> [_]
    timing-out: [_] -> w25
    stop <- _ stop-if-true
    n209 = xnode ("FIFO Method Node")("Timeout"=0) -> ("Element"=w303:u64, "Timed Out?"=w302:bool)  [unwired: 1 in, 1 out]
    n210 = call "HandleFIFOsetting.vi"("timed out"=w302, "Value"=w303) -> ()  [unwired: 10 in]
  }
  n211 = timed-loop {
    timing: w11 -> [_]
    timing-out: [_] -> w10
    stop <- _ stop-if-true
    n212 = xnode ("FIFO Method Node")("Timeout"=0) -> ("Element"=w310:u64, "Timed Out?"=w308:bool)  [unwired: 1 in, 1 out]
    n213 = feedback #21() -> (w309:u64)  [unwired: 1 in]
    n214 = feedback-in #21(w310) -> ()
    n215 = feedback #22() -> (w307:bool)  [unwired: 1 in]
    n216 = feedback-in #22(w308) -> ()
    n217 = call "HandleFeedForward.vi"("timed out"=w307, "Value"=w309) -> ()  [unwired: 10 in]
  }
  n218 = timed-loop {
    timing: w7 -> [_]
    timing-out: [_] -> w6
    shift-right: [w315] -> _
    shift-left: FALSE ("done") -> [w324]
    stop <- _ stop-if-true
    n219 = xnode ("Register Read")() -> ("Data"=w327:bool)  [unwired: 1 in, 1 out]
    n220 = feedback #23() -> (w329:bool)  [unwired: 1 in]
    n221 = call-poly <instrlib>:"Count Down.vi"("count in"=u8 9, "load"=w329, "decrement"=TRUE) -> ("terminal count"=w328:bool)  [unwired: 11 in, 1 out]
    n222 = feedback-in #23(w328) -> ()
    n223 = xnode ("Register Read")() -> ("Data"=w322:u32)  [unwired: 1 in, 1 out]
    n224 = xnode ("Register Read")() -> ("Data"=w319:fxp<+/-,32,2>)  [unwired: 1 in, 1 out]
    n225 = Not(x=w327) -> (.not. x?=w325:bool)
    n226 = xnode ("Register Read")() -> ("Data"=w320:fxp<+/-,32,2>)  [unwired: 1 in, 1 out]
    n227 = xnode ("Register Read")() -> ("Data"=w321:u32)  [unwired: 1 in, 1 out]
    n228 = Or(x=w325, y=w324) -> (x .or. y?=w316:bool)
    n229 = call "Adaptive FF.vi"("Source start addr"=w322, "Reset"=w316, "Destination start addr"=w321, "input valid"=w328, "b0"=w319, "a0"=w320) -> ("done"=w318:bool)  [unwired: 4 in, 1 out]
    n230 = Or(x=w316, y=w318) -> (x .or. y?=w317:bool)
    n231 = call <instrlib>:"Detect Rising Edge.vi"("signal"=w327) -> ("edge detected"=w326:bool)  [unwired: 14 in]
    n232 = Select(t=FALSE ("edge detected"), s=w326, f=w317) -> (s? t:f=w315:bool)
    n233 = Not(x=w315) -> (.not. x?=w314:bool)
    n234 = xnode ("Register Write")("Data"=w314) -> ()  [unwired: 1 in, 1 out]
  }
  n235 = timed-loop {
    timing: w5 -> [_]
    timing-out: [_] -> w4
    shift-right: [w335] -> _
    shift-left: FeedForwardState."Wait for trigger" ("FF state") -> [w344]
    shift-right: [w336] -> _
    shift-left: TRUE ("decrement") -> [w337]
    stop <- _ stop-if-true
    n236 = feedback #24() -> (w341:bool)  [unwired: 1 in]
    n237 = call-poly <instrlib>:"Count Down.vi"("count in"=u8 2, "load"=w341, "decrement"=TRUE) -> ("terminal count"=w340:bool)  [unwired: 11 in, 1 out]
    n238 = feedback-in #24(w340) -> ()
    n239 = call "Adress counter.vi"("input valid"=w340, "Reset"=w337) -> ("output valid"=w339:bool, "Address"=w347:u32)  [unwired: 8 in]
    n240 = feedback #25() -> (w346:u32)  [unwired: 1 in]
    n241 = feedback-in #25(w347) -> ()
    n242 = case shown="\"Read FF\"" w344 {
      selector: w344 -> [w354 w366 w382 w400]
      tunnel: w346 -> [_ _ w379 w397]
      tunnel: [w353 w371 w381 w399] -> w335
      tunnel: "Load FF" -> [w364 w370 _ _]
      tunnel: w339 -> [_ _ w375 _]
      tunnel: "Clear feedback buffers" -> [w360 w369 _ _]
      tunnel: [TRUE ("decrement") TRUE ("decrement") _ _] -> w336
      tunnel: "FF buffers manual" -> [w351 _ _ _]
      frame "Wait for trigger", Default {
        n243 = Select(t=FeedForwardState."Read FF" ("FF state"), s=w364, f=w354) -> (s? t:f=w361:T2)
        n244 = xnode ("Register Write")() -> ("Data"=w357:bool)  [unwired: 1 in, 1 out]
        n245 = xnode ("Register Write")() -> ("Data"=w358:bool)  [unwired: 1 in, 1 out]
        n246 = Select(t=FeedForwardState."Clear FF" ("FF state"), s=w360, f=w361) -> (s? t:f=w355:T2)
        n247 = Not(x=w358) -> (.not. x?=w356:bool)
        n248 = And(x=w357, y=w356) -> (x .and. y?=w352:bool)
        n249 = And(x=w351, y=w352) -> (x .and. y?=w350:bool)
        n250 = call <instrlib>:"Detect Rising Edge.vi"("signal"=w352) -> ("edge detected"=w349:bool)  [unwired: 14 in]
        n251 = Or(x=w350, y=w349) -> (x .or. y?=w348:bool)
        n252 = Select(t=w355, s=w348, f=w354) -> (s? t:f=w353:T2)
      }
      frame "Wait for reset" {
        n253 = Or(x=w369, y=w370) -> (x .or. y?=w368:bool)
        n254 = Select(t=w366, s=w368, f=FeedForwardState."Wait for trigger" ("FF state")) -> (s? t:f=w371:T2)
      }
      frame "Read FF" {
        n255 = xnode ("Memory Method Node")("Address"=w379) -> ("Data"=w390:fxp<+/-,32,14>)  [unwired: 1 in, 1 out]
        n256 = xnode ("Memory Method Node")("Address"=w379) -> ("Data"=w391:fxp<+/-,32,14>)  [unwired: 1 in, 1 out]
        n257 = xnode ("Memory Method Node")("Address"=w379) -> ("Data"=w389:fxp<+/-,32,14>)  [unwired: 1 in, 1 out]
        n258 = xnode ("Memory Method Node")("Address"=w379) -> ("Data"=w380:fxp<+/-,32,14>)  [unwired: 1 in, 1 out]
        n259 = xnode ("Memory Method Node")("Address"=w379) -> ("Data"=w388:fxp<+/-,32,14>)  [unwired: 1 in, 1 out]
        n260 = xnode ("Memory Method Node")("Address"=w379) -> ("Data"=w378:fxp<+/-,32,14>)  [unwired: 1 in, 1 out]
        n261 = feedback #26() -> (w387:fxp<+/-,32,14>)  [unwired: 1 in]
        n262 = feedback-in #26(w390) -> ()
        n263 = feedback #27() -> (w386:fxp<+/-,32,14>)  [unwired: 1 in]
        n264 = feedback-in #27(w389) -> ()
        n265 = feedback #28() -> (w377:fxp<+/-,32,14>)  [unwired: 1 in]
        n266 = feedback-in #28(w380) -> ()
        n267 = feedback #29() -> (w385:fxp<+/-,32,14>)  [unwired: 1 in]
        n268 = feedback-in #29(w388) -> ()
        n269 = feedback #30() -> (w376:fxp<+/-,32,14>)  [unwired: 1 in]
        n270 = feedback-in #30(w378) -> ()
        n271 = feedback #31() -> (w373:fxp<+/-,32,14>)  [unwired: 1 in]
        n272 = feedback-in #31(w391) -> ()
        n273 = xnode ("Register Read")() -> ("Data"=w372:u16)  [unwired: 1 in, 1 out]
        n274 = Build Array(w373, w387, w386, w385, w377, w376) -> (w394:fxp<+/-,32,14>[])
        n275 = call "FormatDMAelement_6_elements.vi"("valid in"=w375, "factor"=w372, "Data in"=w394) -> ("valid out"=w392:bool, "Values"=w393:u64[])  [unwired: 7 in]
        n276 = case shown="True" w392 {
          tunnel: w393 -> [_ w395]
          frame False {
          }
          frame True {
            n277 = xnode ("FIFO Method Node")("Element"=w395, "Timeout"=0) -> ()  [unwired: 1 in, 2 out]
          }
        }
        n278 = Less?(x=w379, y=u32 40000) -> (x < y?=w383:bool)
        n279 = Select(t=w382, s=w383, f=FeedForwardState."Wait for reset" ("FF state")) -> (s? t:f=w381:T2)
      }
      frame "Clear FF" {
        w398 = fxp<+/-,32,14> 0.0 ("Data")
        n280 = xnode ("Memory Method Node")("Address"=w397, "Data"=w398) -> ()  [unwired: 1 in, 1 out]
        n281 = xnode ("Memory Method Node")("Address"=w397, "Data"=w398) -> ()  [unwired: 1 in, 1 out]
        n282 = xnode ("Memory Method Node")("Address"=w397, "Data"=w398) -> ()  [unwired: 1 in, 1 out]
        n283 = xnode ("Memory Method Node")("Address"=w397, "Data"=w398) -> ()  [unwired: 1 in, 1 out]
        n284 = Less?(x=w397, y=u32 40000) -> (x < y?=w402:bool)
        n285 = xnode ("Memory Method Node")("Address"=w397, "Data"=w398) -> ()  [unwired: 1 in, 1 out]
        n286 = xnode ("Memory Method Node")("Address"=w397, "Data"=w398) -> ()  [unwired: 1 in, 1 out]
        n287 = Select(t=w400, s=w402, f=FeedForwardState."Wait for reset" ("FF state")) -> (s? t:f=w399:T2)
      }
    }
  }
  n288 = node-c288(w15) -> ()
  n289 = node-c288(w30) -> ()
  n290 = node-c288(w6) -> ()
  n291 = node-c288(w23) -> ()
  n292 = node-c288(w25) -> ()
  n293 = node-c288(w10) -> ()
  n294 = node-c288(w8) -> ()
  n295 = node-c288(w28) -> ()
  n296 = node-c288(w13) -> ()
  n297 = node-c288(w4) -> ()
  n298 = node-c288() -> (w20:T4)  [unwired: 1 in]
  n299 = timed-loop {
    timing: w20 -> [_]
    timing-out: [_] -> w19
    stop <- _ stop-if-true
    n300 = xnode "FPGA I/O Node"("IO Module\\AO Data Sync"="IO Module\\AO Data Sync") -> ()  [unwired: 1 in, 1 out]
  }
  n301 = node-c288() -> (w22:T4)  [unwired: 1 in]
  n302 = timed-loop {
    timing: w22 -> [_]
    timing-out: [_] -> w21
    stop <- _ stop-if-true
    n303 = xnode "FPGA I/O Node"("IO Module\\SPI Device"="IO Module\\SPI Device", "IO Module\\SPI Address"="IO Module\\SPI Address", "IO Module\\SPI Write Data"="IO Module\\SPI Write Data", "IO Module\\SPI Read"="IO Module\\SPI Read", "IO Module\\SPI Write"="IO Module\\SPI Write") -> ("IO Module\\SPI Idle"=→"IO Module\\SPI Idle":bool, "IO Module\\SPI Read Data"=→"IO Module\\SPI Read Data":u8)  [unwired: 7 in, 7 out]
  }
  n304 = node-c288(w17) -> ()
  n305 = node-c288(w19) -> ()
  n306 = node-c288(w21) -> ()
